vi "Component Reset.vi"(7 "FPGA Interface":refnum<class "FPGA Interface.lvclass">, 8 "error in (no error)":errorcluster, 10 "Component IDs for Reset":u8[](array[numeric]), 11 "1553 Session in":refnum<class "1553 Session.lvclass">) -> (0 "error out":errorcluster, 3 "1553 Session out":refnum<class "1553 Session.lvclass">)   [LabVIEW 2020, in "BCI-1553 API.lvlib" / "1553 Session.lvclass"]
doc: "Performs a full reset of the onboard memory of a target component(s). This should never be called on an active component after it has been configured."
uses:
  1553 Session.lvclass
  Dependencies/FPGA Interface/FPGA Interface.lvclass
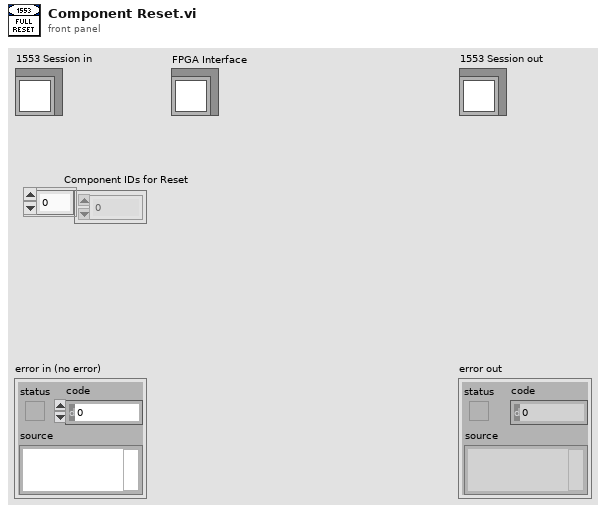
[diagram p1: front panel]
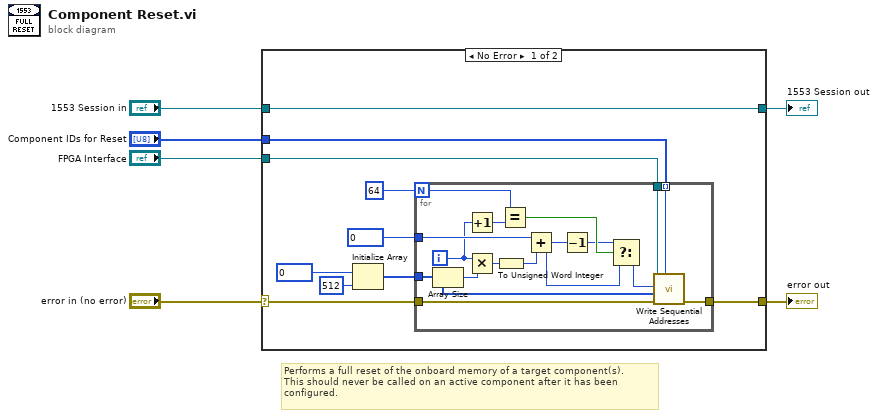
[diagram p0: block diagram]
diagram:
  # "Performs a full reset of the onboard memory of a target component(s).\nThis should never be called on an active component after it has been\nconfigured."
  n1 = case shown="No Error" "error in (no error)" {
    selector: "error in (no error)" -> [w10 w34]
    tunnel: [w9 w34] -> w5
    tunnel: [w16 w33] -> w3
    tunnel: "1553 Session in" -> [w16 w33]
    tunnel: "FPGA Interface" -> [w8 _]
    tunnel: "Component IDs for Reset" -> [w7 _]
    frame No Error {
      n2 = Initialize Array(u16 0 ("Starting Address"), 512 ("dimension size")) -> (w12:u16[])
      n3 = for {
        N: 64 -> [w21]
        tunnel: w8 -> [w32]
        tunnel: w7 -> [w31] mode=indexing
        tunnel: u16 0 ("Starting Address") -> [w25]
        tunnel: w12 -> [w28]
        tunnel: w10 -> [w30]
        tunnel: [w29] -> w9
        i -> [w23]
        n4 = Array Size(array=w28) -> (size(s)=w27:i32)
        n5 = Increment(x=w23) -> (x+1=w22:i32)
        n6 = Multiply(x=w23, y=w27) -> (x*y=w26:i32)
        n7 = To Unsigned Word Integer(number=w26) -> (unsigned 16bit integer=w24:u16)
        n8 = Equal?(x=w21, y=w22) -> (x = y?=w20:bool)
        n9 = Add(x=w25, y=w24) -> (x+y=w18:u16)
        n10 = Decrement(x=w18) -> (x-1=w19:u16)
        n11 = Select(t=w19, s=w20, f=w18) -> (s? t:f=w17:u16)
        n12 = call-dynamic "Write Sequential Addresses.vi"("Target IC (1-8)"=w31, "error in (no error)"=w30, "Data"=w28, "Starting Address"=w17, "FPGA Interface in"=w32) -> ("error out"=w29:errorcluster)  [unwired: 6 in]
      }
    }
    frame Error {
    }
  }
  "error out" <- w5
  "1553 Session out" <- w3
